vi "Get Attribute By ID.vi"(8 "error in (no error)":errorcluster, 10 "ID":i32=-1, 11 "Attributes in":refnum<class "Attributes.lvclass">) -> (0 "error out":errorcluster, 1 "Attribute":refnum<class "Attribute.lvclass">, 3 "Attributes out":refnum<class "Attributes.lvclass">)   [LabVIEW 2019, in "HierDAL Library.lvlib" / "Database.lvlib" / "Repositories.lvlib" / "Attributes.lvclass"]
uses:
  Attributes.lvclass
  Models Library/Attribute Class/Attribute.lvclass
  Attributes.lvclass/Attributes.ctl
  Database Manager Class/Database Manager.lvclass
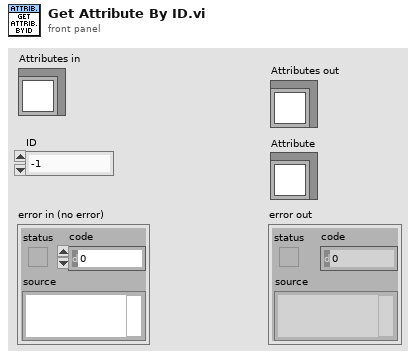
[diagram p1: front panel]
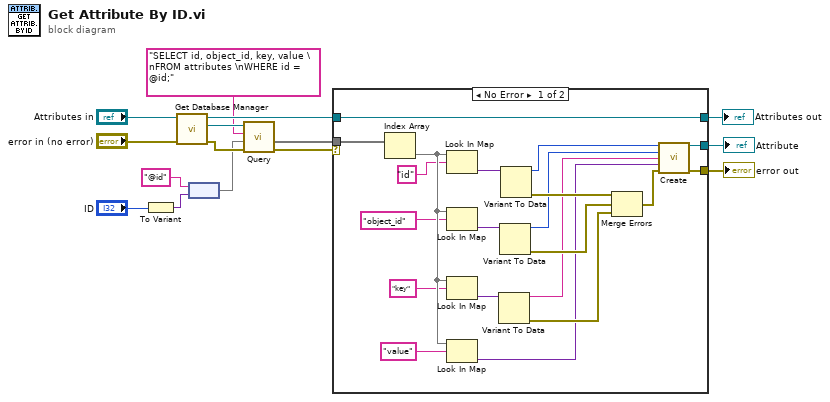
[diagram p0: block diagram]
diagram:
  n1 = To Variant(anything="ID") -> (Variant=w9:variant)
  n2 = call "Get Database Manager.vi"("error in (no error)"="error in (no error)", "Attributes in"="Attributes in") -> ("error out"=w12:errorcluster, "Database Manager"=w13:refnum<class "Database Manager.lvclass">, "Attributes out"=w15:refnum<class "Attributes.lvclass">)  [unwired: 7 in]
  n3 = node("@id" ("key"), w9) -> (w7:map{string, variant})
  n4 = call-dynamic "Query.vi"("error in (no error)"=w12, "Parameters"=w7, "Query"="SELECT id, object_id, key, value \nFROM attributes \nWHERE id = @id;", "Database Manager in"=w13) -> ("error out"=w5:errorcluster, "Rows"=w3:map{string, variant}[])  [unwired: 5 in, 1 out]
  n5 = case shown="No Error" w5 {
    selector: w5 -> [_ w36]
    tunnel: w3 -> [w34 _]
    tunnel: [w26 w36] -> w1
    tunnel: w15 -> [w27 w37]
    tunnel: [w27 w37] -> w4
    tunnel: [w25 _] -> w2
    frame No Error {
      n6 = Index Array(array=w34) -> (element=w35:map{string, variant})  [unwired: 1 in]
      n7 = Look In Map(map=w35, key="id") -> (value=w31:variant)  [unwired: 1 in, 1 out]
      n8 = Look In Map(map=w35, key="object_id") -> (value=w30:variant)  [unwired: 1 in, 1 out]
      n9 = Look In Map(map=w35, key="key") -> (value=w21:variant)  [unwired: 1 in, 1 out]
      n10 = Look In Map(map=w35, key="value") -> (value=w18:variant)  [unwired: 1 in, 1 out]
      n11 = Variant To Data(Variant=w21) -> (data=w19:string, error out=w20:errorcluster)  [unwired: 2 in]
      n12 = Variant To Data(Variant=w30) -> (data=w23:i32, error out=w28:errorcluster)  [unwired: 2 in]
      n13 = Variant To Data(Variant=w31) -> (data=w24:i32, error out=w29:errorcluster)  [unwired: 2 in]
      n14 = Merge Errors(w29, w28, w20) -> (w22:errorcluster)
      n15 = call "Create.vi"("ID"=w24, "Object ID"=w23, "Key"=w19, "Value"=w18, "error in (no error)"=w22) -> ("Attribute out"=w25:refnum<class "Attribute.lvclass">, "error out"=w26:errorcluster)  [unwired: 9 in]
    }
    frame Error {
    }
  }
  "error out" <- w1
  "Attributes out" <- w4
  "Attribute" <- w2
